vi "Construct_Bad_Track_Without_(11-111)_Point-1.vi"(6 "[IN] Indexes for Jumps":i32[](array[numeric]), 8 "error IN":errorcluster, 9 "[IN] Index of recon\nstructed tracks":i32, 10 "[IN] Clusters for Re\nconstructed Tracks":T1, 11 "[IN] Still connected\ntracks in group":T2) -> (0 "error OUT":errorcluster, 2 "[OUT] Clusters for Re\nconstructed Tracks":T1)   [LabVIEW 2013]
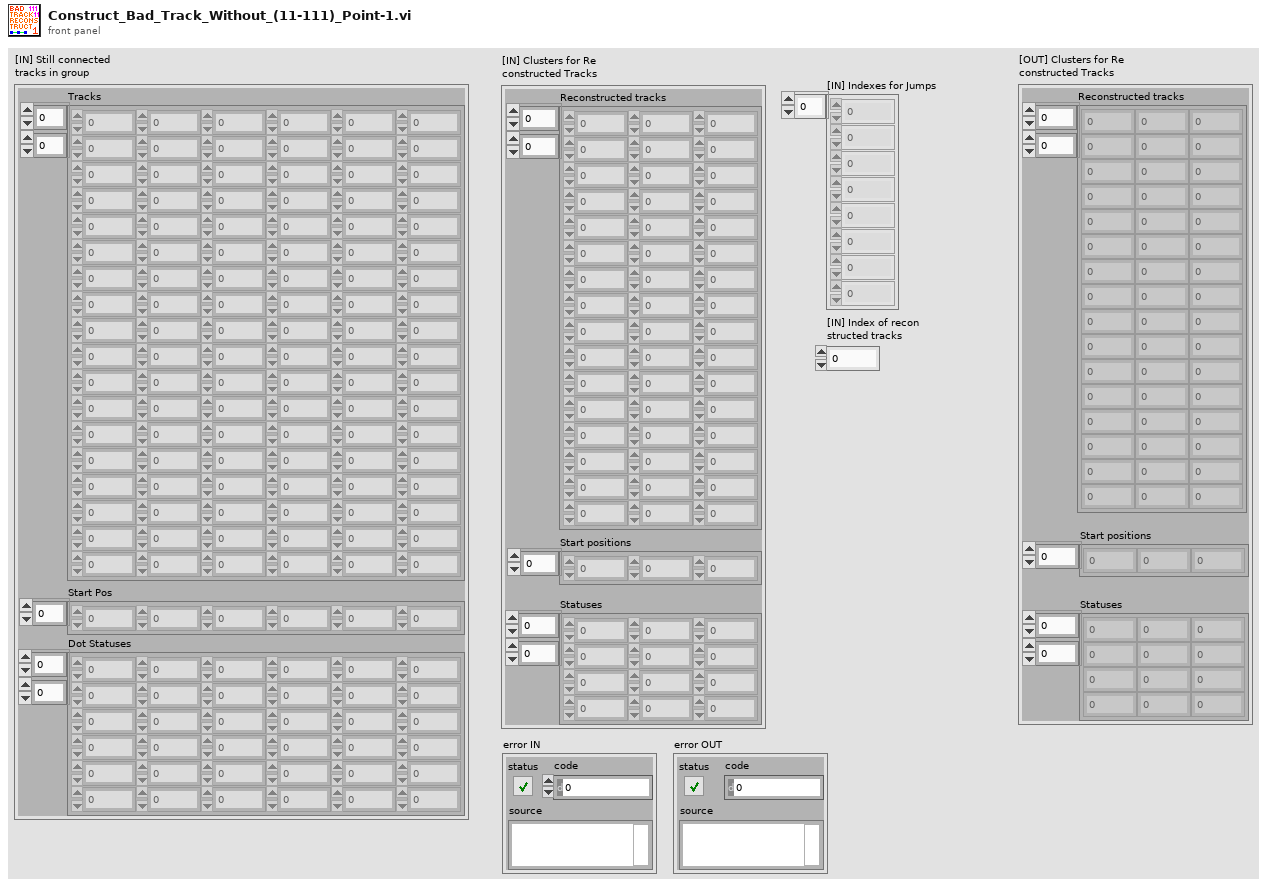
[diagram p1: front panel]
types:
  T1 = cluster{"Reconstructed tracks":dbl[][], "Start positions":i32[], "Statuses":i16[][]}
  T2 = cluster{"Tracks":dbl[][], "Start Pos":i32[], "Dot Statuses":i16[][]}
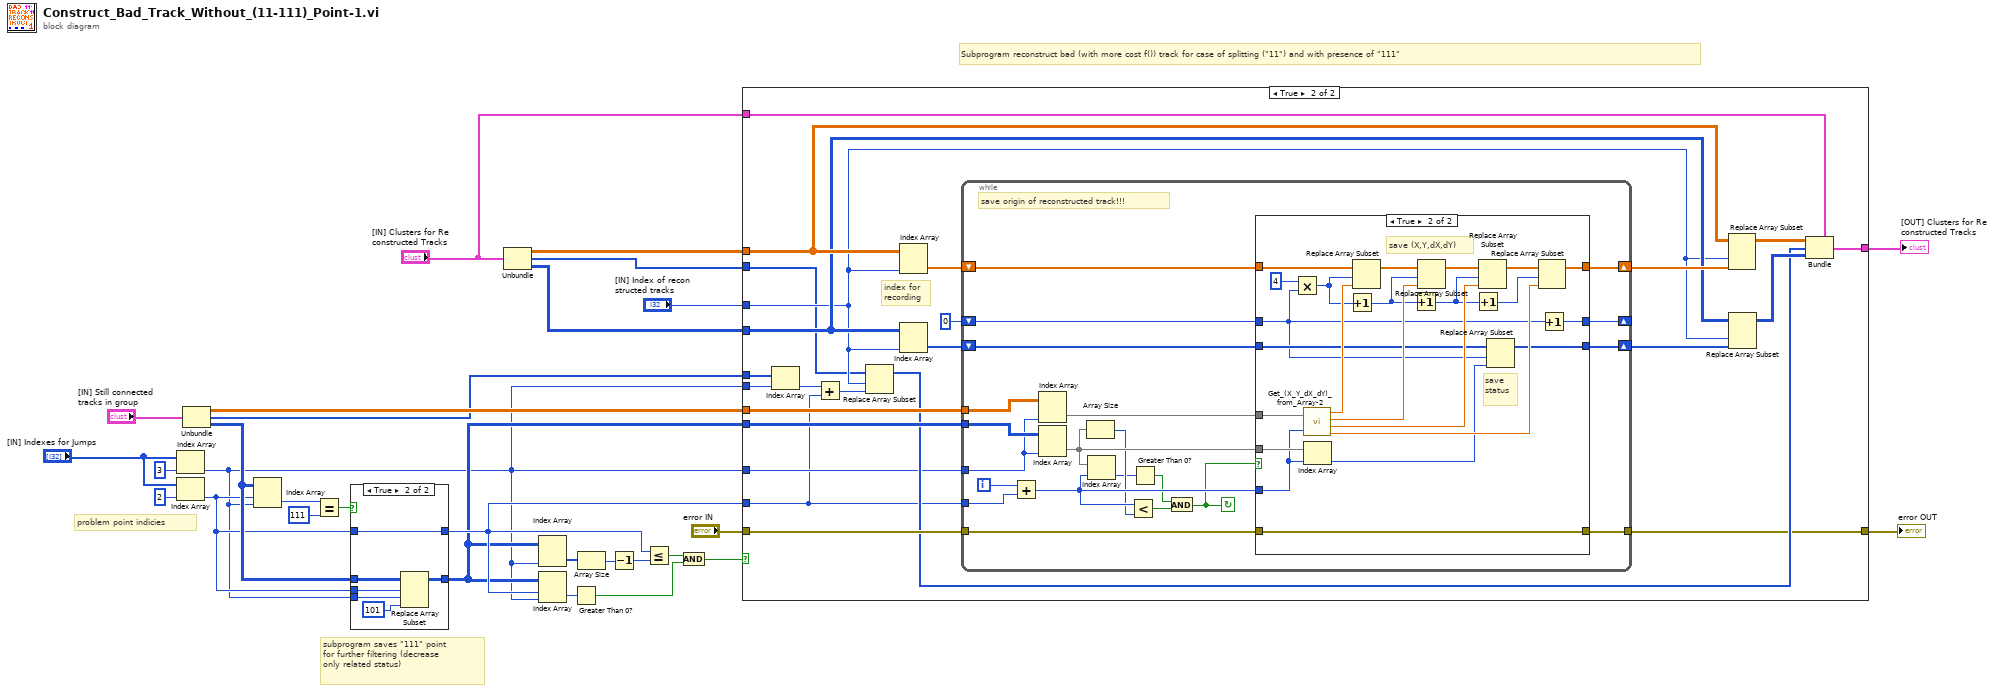
[diagram p0: block diagram]
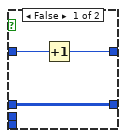
[diagram p2: hidden frame]
diagram:
  # "subprogram saves \"111\" point\nfor further filtering (decrease \nonly related status)"
  # "problem point indicies"
  # "Subprogram reconstruct bad (with more cost f()) track for case of splitting (\"11\") and with presence of \"111\""
  n1 = Index Array(array="[IN] Indexes for Jumps", index=3) -> (element=w1:i32)
  n2 = Index Array(array="[IN] Indexes for Jumps", index=2) -> (element=w2:i32)
  n3 = Unbundle("[IN] Still connected\ntracks in group") -> ("Tracks"=w25:dbl[][], "Start Pos"=w10:i32[], "Dot Statuses"=w4:i16[][])
  n4 = Index Array(array=w4, index (row)=w2, index (col)=w1) -> (element=w7:i16)
  n5 = Equal?(x=w7, y=i16 111) -> (x = y?=w6:bool)
  n6 = case shown="True" w6 {
    tunnel: w2 -> [w32 w38]
    tunnel: [w31 w38] -> w5
    tunnel: w4 -> [w30 w37]
    tunnel: [w30 w36] -> w3
    tunnel: w2 -> [_ w35]
    tunnel: w1 -> [_ w34]
    frame False {
      n7 = Increment(x=w32) -> (x+1=w31:i32)
    }
    frame True {
      n8 = Replace Array Subset(array=w37, new element=i16 101 ("new element/subarray"), index (row)=w35, index (col)=w34) -> (w36:i16[][])
    }
  }
  n9 = Unbundle("[IN] Clusters for Re\nconstructed Tracks") -> ("Reconstructed tracks"=w24:dbl[][], "Start positions"=w9:i32[], "Statuses"=w23:i16[][])
  n10 = Index Array(array=w3, index (col)=w1) -> (element=w19:i16[])  [unwired: 1 in]
  n11 = Index Array(array=w3, index (row)=w5, index (col)=w1) -> (element=w20:i16)
  n12 = Greater Than 0?(x=w20) -> (x > 0?=w15:bool)
  n13 = Array Size(array=w19) -> (size(s)=w18:i32)
  n14 = Decrement(x=w18) -> (x-1=w17:i32)
  n15 = Less Or Equal?(x=w5, y=w17) -> (x <= y?=w16:bool)
  n16 = And(x=w16, y=w15) -> (x .and. y?=w14:bool)
  n17 = case shown="True" w14 {
    tunnel: w25 -> [_ w61]
    tunnel: w24 -> [_ w54]
    tunnel: w23 -> [_ w53]
    tunnel: "[IN] Index of recon\nstructed tracks" -> [_ w48]
    tunnel: "error IN" -> [w39 w60]
    tunnel: w3 -> [_ w59]
    tunnel: "[IN] Clusters for Re\nconstructed Tracks" -> [w40 w55]
    tunnel: w10 -> [_ w49]
    tunnel: w1 -> [_ w51]
    tunnel: w5 -> [_ w43]
    tunnel: [w40 w45] -> w11
    tunnel: w1 -> [_ w44]
    tunnel: [w39 w42] -> w12
    tunnel: w9 -> [_ w41]
    frame False {
    }
    frame True {
      # "index for\nrecording"
      n18 = Index Array(array=w49, index=w51) -> (element=w50:i32)
      n19 = Add(x=w50, y=w43) -> (x+y=w47:i32)
      n20 = Replace Array Subset(array=w41, new element=w47, index=w48) -> (w46:i32[])
      n21 = Index Array(array=w54, index (col)=w48) -> (element=w64:dbl[])  [unwired: 1 in]
      n22 = Index Array(array=w53, index (col)=w48) -> (element=w63:i16[])  [unwired: 1 in]
      n23 = while {
        tunnel: w43 -> [w72]
        tunnel: w61 -> [w85]
        tunnel: w59 -> [w84]
        tunnel: w44 -> [w83]
        shift-right: [w78] -> w56
        shift-left: w64 -> [w82]
        shift-right: [w76] -> w52
        shift-left: w63 -> [w80]
        shift-right: [w77] -> _
        shift-left: 0 -> [w79]
        tunnel: w60 -> [w75]
        tunnel: [w74] -> w42
        i -> [w73]
        stop <- w65 continue-if-true
        # "save origin of reconstructed track!!!"
        n24 = Add(x=w73, y=w72) -> (x+y=w71:i32)
        n25 = Index Array(array=w85, index (col)=w83) -> (element=w81:dbl[])  [unwired: 1 in]
        n26 = Index Array(array=w84, index (col)=w83) -> (element=w70:i16[])  [unwired: 1 in]
        n27 = Array Size(array=w70) -> (size(s)=w69:i32)
        n28 = Index Array(array=w70, index=w71) -> (element=w67:i16)
        n29 = Less?(x=w71, y=w69) -> (x < y?=w66:bool)
        n30 = Greater Than 0?(x=w67) -> (x > 0?=w68:bool)
        n31 = And(x=w68, y=w66) -> (x .and. y?=w65:bool)
        n32 = case shown="True" w65 {
          tunnel: w82 -> [w89 w110]
          tunnel: w81 -> [_ w112]
          tunnel: w70 -> [_ w111]
          tunnel: w71 -> [_ w95]
          tunnel: w80 -> [w87 w97]
          tunnel: [w87 w94] -> w76
          tunnel: [w89 w93] -> w78
          tunnel: w79 -> [w88 w92]
          tunnel: [w88 w91] -> w77
          tunnel: w75 -> [w86 w90]
          tunnel: [w86 w90] -> w74
          frame False {
          }
          frame True {
            # "save (X,Y,dX,dY)"
            # "save\nstatus"
            n33 = Multiply(x=4, y=w92) -> (x*y=w106:i32)
            n34 = call "Get_(X_Y_dX_dY)_from_Array-2.vi"("(X,Y,dX,dY)"=w112, "Index of Displacement"=w95) -> ("X"=w108:dbl, "Y"=w105:dbl, "dX"=w102:dbl, "dY"=w98:dbl)
            n35 = Index Array(array=w111, index=w95) -> (element=w96:i16)
            n36 = Increment(x=w106) -> (x+1=w103:i32)
            n37 = Replace Array Subset(array=w110, new element=w108, index=w106) -> (w107:dbl[])
            n38 = Increment(x=w103) -> (x+1=w101:i32)
            n39 = Replace Array Subset(array=w107, new element=w105, index=w103) -> (w104:dbl[])
            n40 = Increment(x=w101) -> (x+1=w100:i32)
            n41 = Replace Array Subset(array=w104, new element=w102, index=w101) -> (w99:dbl[])
            n42 = Replace Array Subset(array=w97, new element=w96, index=w92) -> (w94:i16[])
            n43 = Replace Array Subset(array=w99, new element=w98, index=w100) -> (w93:dbl[])
            n44 = Increment(x=w92) -> (x+1=w91:i32)
          }
        }
      }
      n45 = Replace Array Subset(array=w54, new element=w56, index (col)=w48) -> (w57:dbl[][])  [unwired: 1 in]
      n46 = Replace Array Subset(array=w53, new element=w52, index (col)=w48) -> (w58:i16[][])  [unwired: 1 in]
      n47 = Bundle(cluster=w55, "Reconstructed tracks"=w57, "Start positions"=w46, "Statuses"=w58) -> (w45:T1)
    }
  }
  "[OUT] Clusters for Re\nconstructed Tracks" <- w11
  "error OUT" <- w12
